vi "get array from cxd.vi"(8 "error in (no error)":errorcluster, 10 "Image file path":path, 11 "Autofocus in":refnum<class "Autofocus.lvclass">) -> (0 "error out":errorcluster, 3 "Autofocus out":refnum<class "Autofocus.lvclass">)   [LabVIEW 2012, in "Autofocus.lvclass"]
uses:
  Autofocus.lvclass
  Autofocus.lvclass/Autofocus.ctl
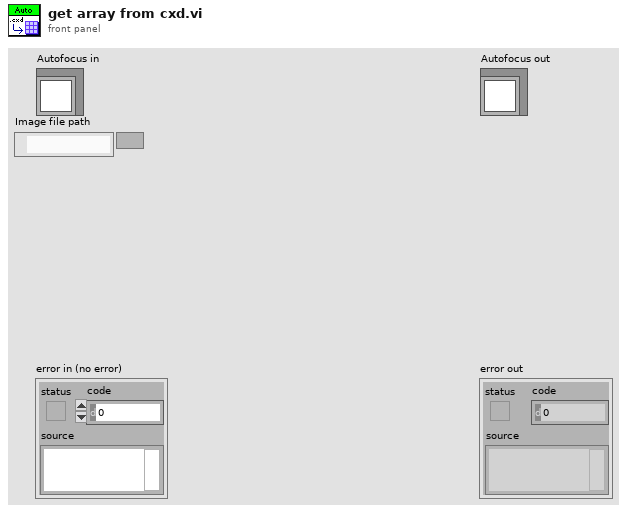
[diagram p1: front panel]
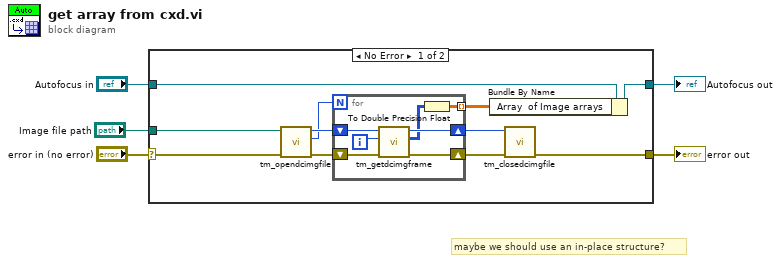
[diagram p0: block diagram]
diagram:
  # "maybe we should use an in-place structure?"
  n1 = case shown="No Error" "error in (no error)" {
    selector: "error in (no error)" -> [w16 w24]
    tunnel: [w8 w24] -> w2
    tunnel: [w12 w25] -> w3
    tunnel: "Autofocus in" -> [w13 w25]
    tunnel: "Image file path" -> [w6 _]
    frame No Error {
      n2 = call <userlib>:"tm_opendcimgfile.vi"("error in (no error)"=w16, "Path"=w6) -> ("error out"=w15:errorcluster, "Total Frames"=w11:i32, "File Handle"=w14:u32)  [unwired: 7 in]
      n3 = for {
        N: w11 -> [_]
        tunnel: [w19] -> w10 mode=indexing
        shift-right: [w21] -> w9
        shift-left: w15 -> [w23]
        shift-right: [w20] -> w7
        shift-left: w14 -> [w22]
        i -> [w17]
        n4 = call <userlib>:"tm_getdcimgframe.vi"("error in (no error)"=w23, "Frame Index"=w17, "File Handle in"=w22) -> ("error out"=w21:errorcluster, "Data"=w18:u16[][], "File Handle out"=w20:u32)  [unwired: 5 in, 1 out]
        n5 = To Double Precision Float(number=w18) -> (double precision float=w19:dbl[][])
      }
      n6 = Bundle By Name(cluster=w13, "Array  of Image arrays"=w10) -> (w12:refnum<class "Autofocus.lvclass">)
      n7 = call <userlib>:"tm_closedcimgfile.vi"("error in (no error)"=w9, "File Handle"=w7) -> ("error out"=w8:errorcluster)  [unwired: 9 in]
    }
    frame Error {
    }
  }
  "error out" <- w2
  "Autofocus out" <- w3
